vi "GENERTOR.vi"() -> ()   [LabVIEW 2025]
panel:
  out "Send command 2":string
  in  "Modulating Depth (%)":dbl(knob) min=0.0 max=120.0 step=1.0 scale=0.0..120.0
  in  "Frequency units 2":u32(ring) items=["Hz"=1, "KHz"=1000, "MHz"=1000000]
  in  "Signal source":bool
  in  "Waveform 2":u16(ring) items=["SIN", "SQU", "TRI", "RAMP", "USER"]
  in  "Modulating Frequency":dbl(knob) min=0.0 max=1000.0 step=1.0 scale=2.0..1000.0
  out "Send command":string
  in  "stop":bool
  in  "AM":bool
  in  "Address":u8
  in  "Frequency units":u32(ring) items=["Hz"=1, "KHz"=1000, "MHz"=1000000]
  in  "Offset":dbl(knob) min=0.0 max=50.0 step=0.1 scale=0.0..50.0
  in  "Frequency":dbl(knob) min=0.0 max=1000.0 step=1.0 scale=2.0..1000.0
  in  "Waveform":u16(ring) items=["SIN", "SQU", "TRI", "RAMP", "NOI", "DC", "USER"]
  in  "Amplitude":dbl(knob)=0.1 min=0.1 max=10.0 step=0.1 scale=0.1..10.0
  # "External"
  # "Both"
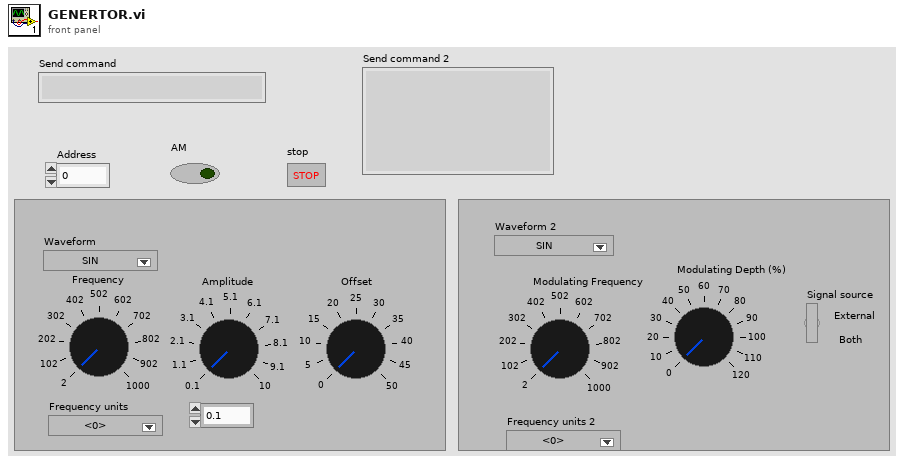
[diagram p1: front panel]
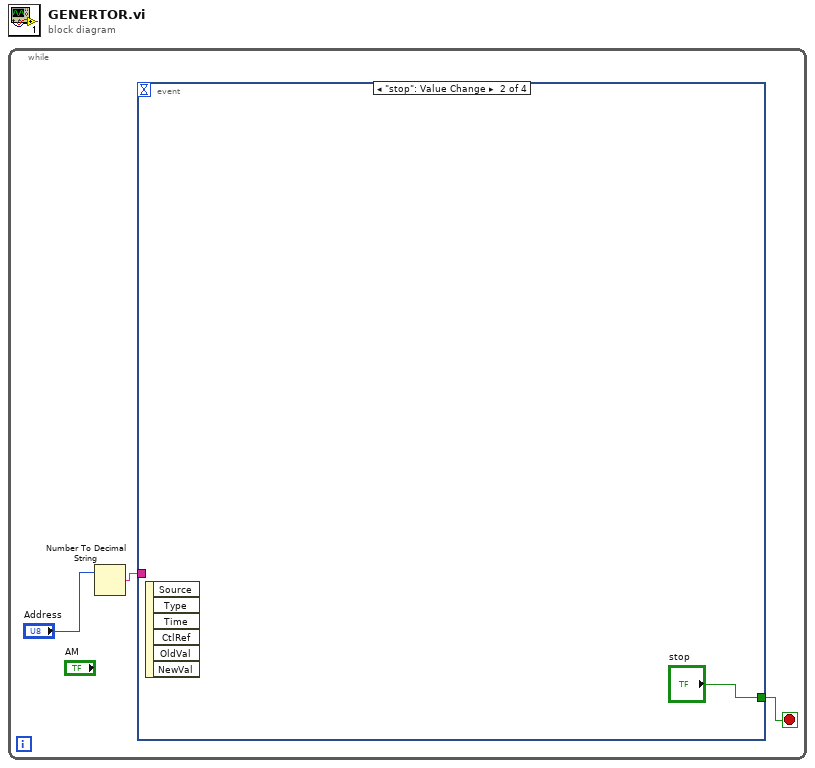
[diagram p0: block diagram]
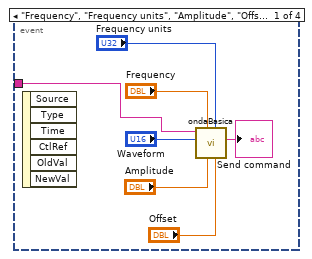
[diagram p2: hidden frame]
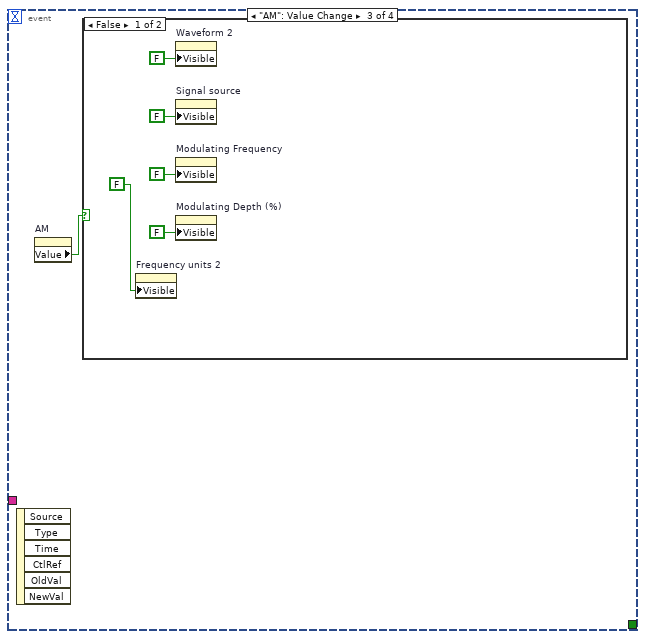
[diagram p3: hidden frame]
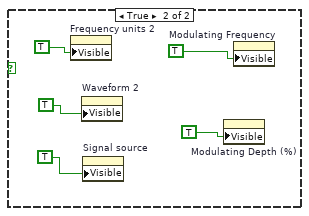
[diagram p4: hidden frame]
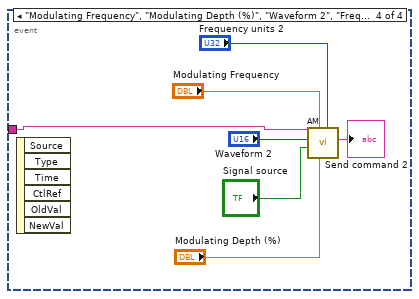
[diagram p5: hidden frame]
diagram:
  n1 = while {
    stop <- w1 stop-if-true
    n2 = Number To Decimal String(number="Address") -> (decimal integer string=w2:string)  [unwired: 1 in]
    n3 = event shown="[1] \"stop\": Value Change" {
      selector: _ -> [_ _ _ _]
      dyn-events: _ -> [_ _ _ _]
      timeout: _ -> [_ _ _ _]
      tunnel: w2 -> [w5 _ _ w23]
      tunnel: [_ "stop" _ _] -> w1
      event "Frequency", "Frequency units", "Amplitude", "Offset": Value Change {
        n4 = event-data() -> ()  [unwired: 1 in, 6 out]
        n5 = call "ondaBasica.vi"("Offset"="Offset", "Frequency units"="Frequency units", "Amplitude"="Amplitude", "Frequency"="Frequency", "Waveform"="Waveform", "Address"=w5) -> ("Send command"=→"Send command":string)  [unwired: 3 in, 2 out]
      }
      event "stop": Value Change {
        n6 = event-data() -> ()  [unwired: 1 in, 6 out]
      }
      event "AM": Value Change {
        n7 = event-data() -> ()  [unwired: 1 in, 6 out]
        n8 = property on="AM" class="Bool (strict)"() -> ("Value"=w12:bool)  [unwired: 2 in, 2 out]
        n9 = case shown="False" w12 {
          frame False {
            n10 = property on="Frequency units 2" class="Ring (strict)"("Visible"=FALSE) -> ()  [unwired: 2 in, 2 out]
            n11 = property on="Waveform 2" class="Ring (strict)"("Visible"=FALSE) -> ()  [unwired: 2 in, 2 out]
            n12 = property on="Signal source" class="Bool (strict)"("Visible"=FALSE) -> ()  [unwired: 2 in, 2 out]
            n13 = property on="Modulating Frequency" class="Knob (strict)"("Visible"=FALSE) -> ()  [unwired: 2 in, 2 out]
            n14 = property on="Modulating Depth (%)" class="Knob (strict)"("Visible"=FALSE) -> ()  [unwired: 2 in, 2 out]
          }
          frame True {
            n15 = property on="Frequency units 2" class="Ring (strict)"("Visible"=TRUE) -> ()  [unwired: 2 in, 2 out]
            n16 = property on="Waveform 2" class="Ring (strict)"("Visible"=TRUE) -> ()  [unwired: 2 in, 2 out]
            n17 = property on="Signal source" class="Bool (strict)"("Visible"=TRUE) -> ()  [unwired: 2 in, 2 out]
            n18 = property on="Modulating Depth (%)" class="Knob (strict)"("Visible"=TRUE) -> ()  [unwired: 2 in, 2 out]
            n19 = property on="Modulating Frequency" class="Knob (strict)"("Visible"=TRUE) -> ()  [unwired: 2 in, 2 out]
          }
        }
      }
      event "Modulating Frequency", "Modulating Depth (%)", "Waveform 2", "Frequency units 2", "Signal source": Value Change {
        n20 = event-data() -> ()  [unwired: 1 in, 6 out]
        n21 = call "AM.vi"("Frequency units"="Frequency units 2", "Modulating Depth (%)"="Modulating Depth (%)", "Modulating Frequency"="Modulating Frequency", "Signal source"="Signal source", "Waveform"="Waveform 2", "Address"=w23) -> ("Send command"=→"Send command 2":string)  [unwired: 3 in, 2 out]
      }
    }
  }
